vi "CAN Messwerte.vi"() -> (1 "CAN data":T1[](array[typedef]) {"payload" format="%x"; "timestamp" format="%<%.7X\n%x>T"; "type" items=["CAN Data"=0, "CAN Remote"=1, "CAN Bus Error"=2, "CAN 2.0 Data"=8, "CAN FD Data"=16, "CAN FD+BRS Data"=24, "J1939 Data"=192, "Delay"=224, "Log Trigger"=225, "Start Trigger"=226]; "identifier" format="%x"})   [LabVIEW 2020, in "CAN Interface.lvlib"]
uses:
  CAN Interface.lvlib
  <vilib>/xnet/xnet.llb/XNET Frame CAN.ctl
  <vilib>/xnet/xnet.llb/XNET Frame Type CAN.ctl
  FGV CAN Daten Aktionen.ctl
  Stoermeldungen/FGV Stoerungen Aktionen.ctl
  Allgemein/FGV Zustaende Aktionen.ctl
  Allgemein/FGV FT-IR Kuehlung Aktionen.ctl
  Stoermeldungen/Stoermeldungen.lvlib
  Allgemein/Allgemein.lvlib
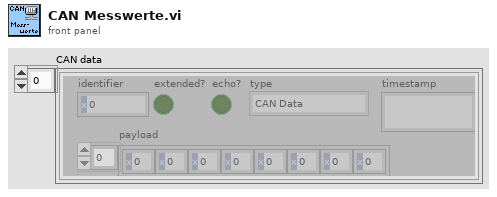
[diagram p1: front panel]
types:
  T1 = typedef "XNET Frame CAN.ctl" = cluster{"timestamp":timestamp, "payload":u8[], "identifier":u32, "type":T2, "extended?":bool, "echo?":bool}
  T2 = typedef "XNET Frame Type CAN.ctl" = u8
  T3 = typedef "Allgemein.lvlib/FGV FT-IR Kuehlung Aktionen.ctl" = enum16{"lesen", "Kühlung?"}
  T4 = typedef "Allgemein.lvlib/FGV Zustaende Aktionen.ctl" = enum16{"lesen", "Zustand PC", "Zustand cRIO", "Bildnummer", "Samplepoint", "Sysloglevel"}
  T5 = typedef "Stoermeldungen.lvlib/FGV Stoerungen Aktionen.ctl" = enum16{"lesen", "Störung aktiv?", "1-64", "65-128"}
  T6 = typedef "CAN Interface.lvlib/FGV CAN Daten Aktionen.ctl" = enum16{"lesen", "Daten", "Konfig", "laden", "speichern", "Status"}
  T7 = typedef "Funktionstasten.lvlib/Zustaende.ctl" = enum16{"Standby", "Pause", "Eco", "Messen", "Kalibrieren", "Spülen Filter", "Spülen Leitung", "Umgebungsluft", "0-Gas", "Cal-Gas", "CG zu PNS", "-------------", "Init 1", "Init 2", "Init 3", "Init 4", "Messen vorbereiten", "Messen durchführen", "Exit"}
  T8 = typedef "CAN Konfig.lvlib/Konfig Daten PC.ctl" = cluster{"Baude Rate":T9, "COM state":u8, "Frame-ID FTIR Start":u32, "Frame-ID FTIR End":u32, "Frame-ID Status Start":u32, "Frame-ID Status End":u32, "Zustand Information":u32, "Aktion":u32, "Frame-ID FTIR Arry":u32[], "Frame-ID Status Arry":u32[], "GPS Start":u32, "Interface":refnum<k21>}
  T9 = typedef "CAN Interface.lvlib/Baude Rate.ctl" = u32
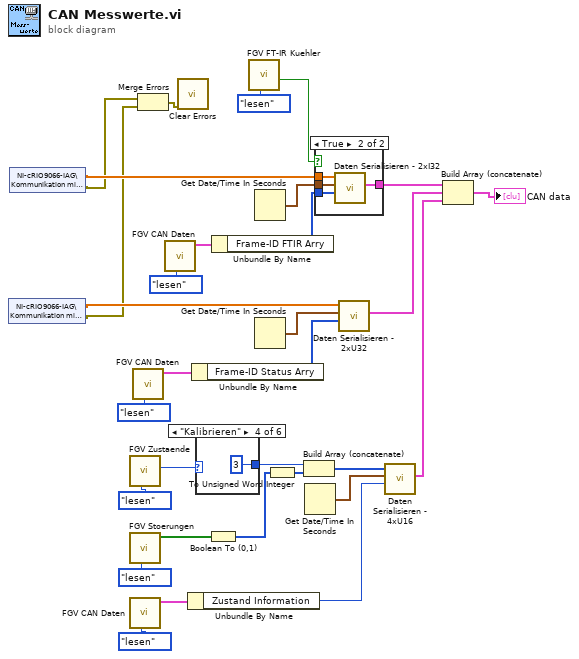
[diagram p0: block diagram]
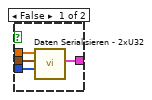
[diagram p2: hidden frame]
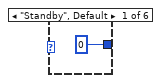
[diagram p3: hidden frame]
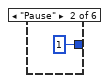
[diagram p4: hidden frame]
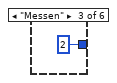
[diagram p5: hidden frame]
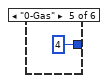
[diagram p6: hidden frame]
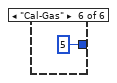
[diagram p7: hidden frame]
diagram:
  n1 = shared-variable "NI-cRIO9066-IAG\\Kommunikation mit PC.lvlib\\Status"() -> (w2:sgl[], error out=w1:errorcluster)  [unwired: 1 in]
  n2 = shared-variable "NI-cRIO9066-IAG\\Kommunikation mit PC.lvlib\\FTIR 1"() -> (w4:sgl[], error out=w3:errorcluster)  [unwired: 1 in]
  n3 = call "FGV Zustaende.vi"("Aktionen"=FGV_Zustaende_Aktionen."lesen") -> ("Zustand cRIO"=w14:T7)  [unwired: 6 in, 4 out]
  n4 = call "FGV Stoerungen.vi"("Aktionen"=FGV_Stoerungen_Aktionen."lesen") -> ("Störung aktiv?"=w16:bool[])  [unwired: 8 in, 2 out]
  n5 = call "FGV CAN Daten.vi"("Aktionen"=FGV_CAN_Daten_Aktionen."lesen") -> ("Konfig Daten"=w19:T8)  [unwired: 8 in, 2 out]
  n6 = call "FGV CAN Daten.vi"("Aktionen"=FGV_CAN_Daten_Aktionen."lesen") -> ("Konfig Daten"=w24:T8)  [unwired: 8 in, 2 out]
  n7 = Merge Errors(w3, w1) -> (w20:errorcluster)
  n8 = call "FGV CAN Daten.vi"("Aktionen"=FGV_CAN_Daten_Aktionen."lesen") -> ("Konfig Daten"=w30:T8)  [unwired: 8 in, 2 out]
  n9 = call <vilib>:"Clear Errors.vi"("error in (no error)"=w20) -> ()  [unwired: 5 in, 2 out]
  n10 = Unbundle By Name(w19) -> ("Zustand Information"=w8:u32)
  n11 = Unbundle By Name(w24) -> ("Frame-ID Status Arry"=w23:u32[])
  n12 = case shown="\"Kalibrieren\"" w14 {
    tunnel: [u16 0 u16 1 u16 2 u16 3 u16 4 u16 5] -> w13
    frame "Standby", Default {
    }
    frame "Pause" {
    }
    frame "Messen" {
    }
    frame "Kalibrieren" {
    }
    frame "0-Gas" {
    }
    frame "Cal-Gas" {
    }
  }
  n13 = Boolean To (0,1)(Boolean=w16) -> (0, 1=w11:i16[])
  n14 = Unbundle By Name(w30) -> ("Frame-ID FTIR Arry"=w29:u32[])
  n15 = call "FGV FT-IR Kuehler.vi"("Aktionen"=FGV_FT-IR_Kuehlung_Aktionen."lesen") -> ("Durchflusssensor 0-5V"=w5:bool)  [unwired: 6 in, 4 out]
  n16 = Get Date/Time In Seconds() -> (seconds since 1Jan1904=w28:timestamp)
  n17 = Get Date/Time In Seconds() -> (seconds since 1Jan1904=w22:timestamp)
  n18 = To Unsigned Word Integer(number=w11) -> (unsigned 16bit integer=w12:u16[])
  n19 = Build Array (concatenate)(w13, w12) -> (w10:u16[])
  n20 = Get Date/Time In Seconds() -> (seconds since 1Jan1904=w9:timestamp)
  n21 = case shown="True" w5 {
    tunnel: w29 -> [w41 w45]
    tunnel: w28 -> [w40 w44]
    tunnel: [w39 w43] -> w27
    tunnel: w4 -> [w38 w42]
    frame False {
      n22 = call "Daten Serialisieren - 2xU32.vi"("Frame-ID"=w41, "Aktuelle Zeit"=w40, "Messdaten"=w38) -> ("data"=w39:T1[])  [unwired: 8 in]
    }
    frame True {
      n23 = call "Daten Serialisieren - 2xI32.vi"("Frame-ID"=w45, "Aktuelle Zeit"=w44, "Messdaten"=w42) -> ("data"=w43:T1[])  [unwired: 8 in]
    }
  }
  n24 = call "Daten Serialisieren - 2xU32.vi"("Frame-ID"=w23, "Aktuelle Zeit"=w22, "Messdaten"=w2) -> ("data"=w21:T1[])  [unwired: 8 in]
  n25 = call "Daten Serialisieren - 4xU16.vi"("Frame-ID"=w8, "Aktuelle Zeit"=w9, "Messdaten"=w10) -> ("data"=w7:T1[])  [unwired: 7 in, 1 out]
  n26 = Build Array (concatenate)(w27, w21, w7) -> (→"CAN data":T1[])
